vi "Nano-Drive Attached.vi"(1 "Handle":i32) -> (0 "DeviceAttached":bool)   [LabVIEW 2012]
uses:
  Madlib.dll
panel:
  # "This VI waits a configurable period of time (10 ms by default) and\nthen returns true/false depending on whether or not a Nano-Drive\nis attached."
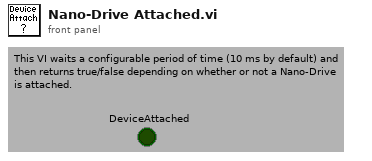
[diagram p1: front panel]
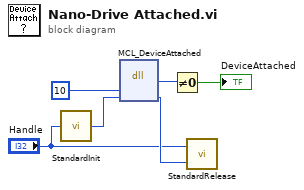
[diagram p0: block diagram]
diagram:
  n1 = call "StandardInit.vi"("Incoming Handle"="Handle") -> ("Outgoing Handle"=w3:i32)
  n2 = dll-call lib="C:/Users/Labview/Desktop/SRR/Madlib_x64/Labview Examples/MADLib.dll" fn="MCL_DeviceAttached"("milliseconds"=10, "handle"=w3) -> (w5:u8, "handle"=w2:i32)  [unwired: 4 in, 2 out]
  n3 = Not Equal To 0?(x=w5) -> (x != 0?=→"DeviceAttached":bool)
  n4 = call "StandardRelease.vi"("Outgoing Handle"=w2, "Incoming Handle"="Handle") -> ()  [unwired: 1 in]
